vi "Errors Handle Dialoge.vi"(4 ">0, AutoClose":u32, 5 "VI Ref":refnum<vi>, 6 "Cancel Text":string="Cancel", 7 "OK Text":string="OK", 8 "error in (no error)":errorcluster, 9 "DisplayDialog":bool, 10 "Title Text":string, 11 "Message":string="\n\r") -> (0 "error out":errorcluster, 2 "OK?":bool=TRUE)   [LabVIEW 2021]
doc: "Name: 蒋松\nEmail: jiangsong@outlook.com"
uses:
  <userlib>/sushu/Tools/Front Panel State.ctl
panel:
  in  "CloseCounter":string
  in  "Cancel":bool
  in  "OK":bool
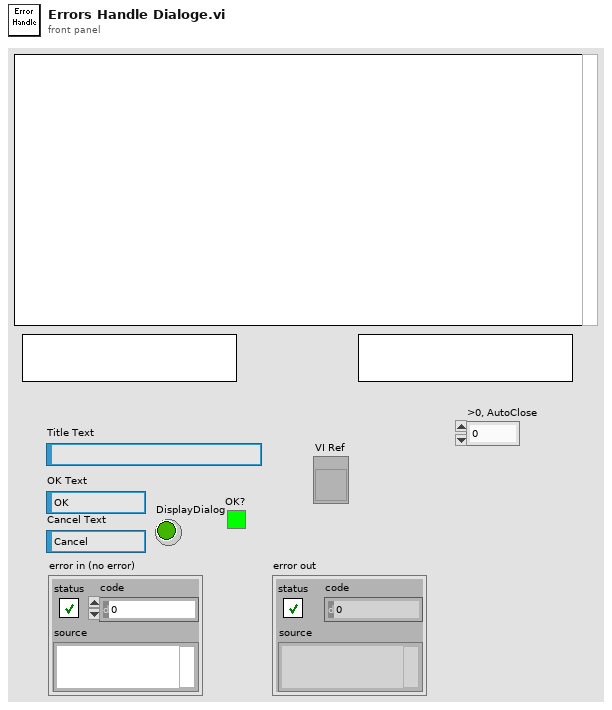
[diagram p1: front panel]
types:
  T1 = typedef "Front Panel State.ctl" = string
  T2 = enum32{"Invalid", "Default", "Floating", "Floating/Auto-Hide", "Modal"}
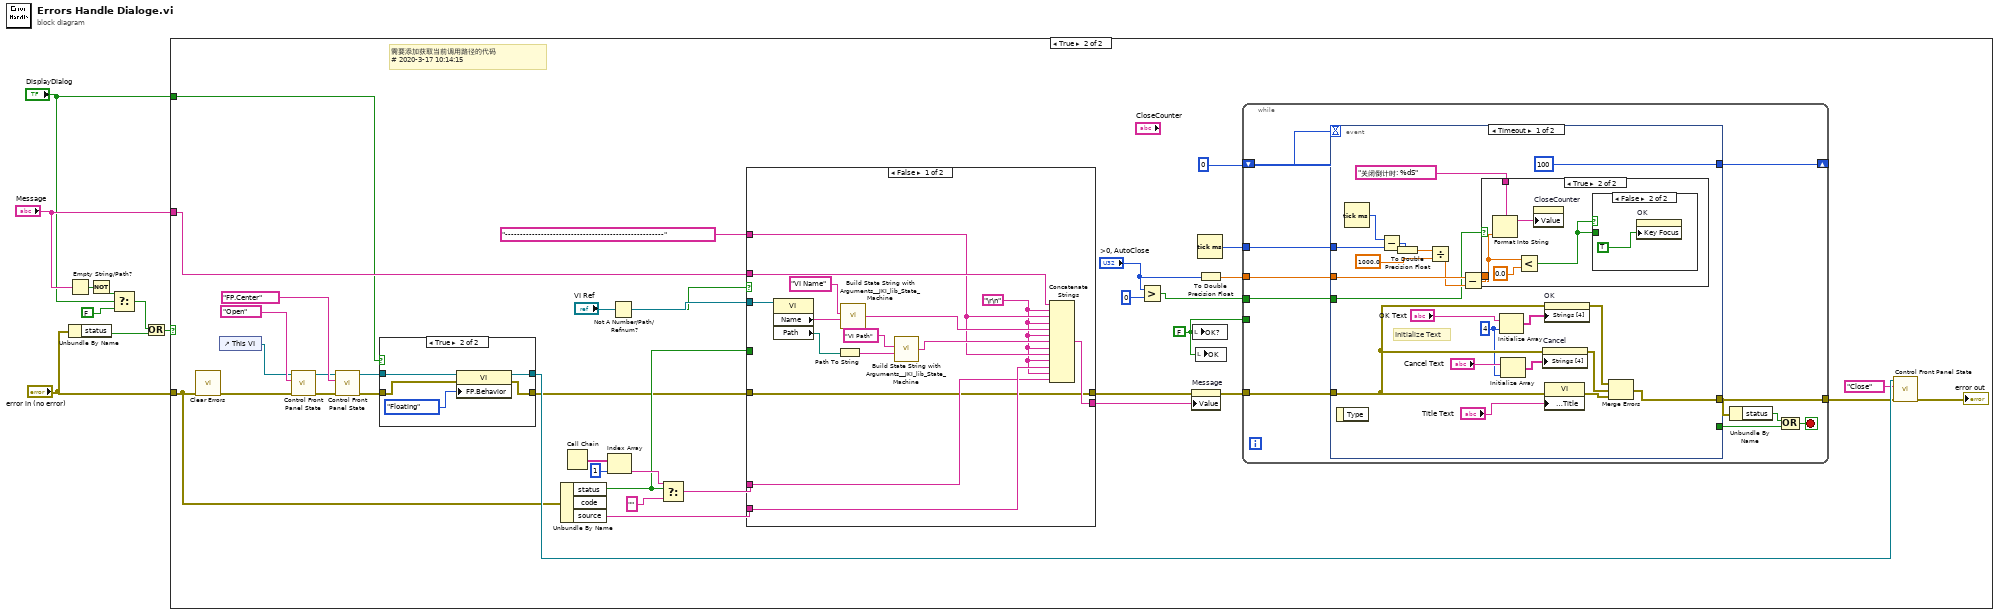
[diagram p0: block diagram]
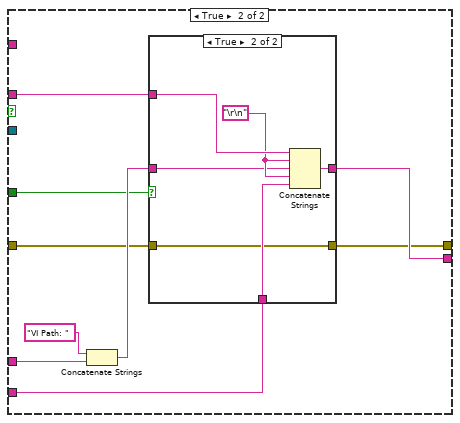
[diagram p4: hidden frame]
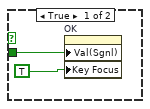
[diagram p7: hidden frame]
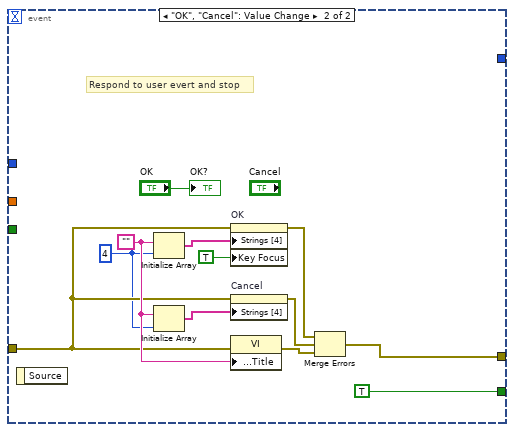
[diagram p8: hidden frame]
diagram:
  n1 = Empty String/Path?(string/path="Message") -> (empty?=w5:bool)
  n2 = Unbundle By Name("error in (no error)") -> ("status"=w9:bool)
  n3 = Not(x=w5) -> (.not. x?=w3:bool)
  n4 = Select(t=w3, s="DisplayDialog", f=FALSE) -> (s? t:f=w4:bool)
  n5 = Or(x=w4, y=w9) -> (x .or. y?=w8:bool)
  n6 = case shown="True" w8 {
    tunnel: "error in (no error)" -> [_ w29]
    tunnel: "Message" -> [_ w34]
    tunnel: "DisplayDialog" -> [_ w30]
    frame False {
    }
    frame True {
      w11 = FALSE ("OK?")
      # "需要添加获取当前调用路径的代码\n# 2020-3-17 10:14:15"
      n7 = call <vilib>:"Clear Errors.vi"("error in (no error)"=w29) -> ("error out"=w28:errorcluster)  [unwired: 5 in, 1 out]
      n8 = control-ref of="This VI"() -> (w26:refnum<vi>)
      n9 = call <userlib>:"Control Front Panel State.vi"("error out"=w28, "Argument"=T1 "Open", "Core.Current VI Reference"=w26) -> ("error out"=w40:errorcluster, "reference out"=w27:refnum<vi>)  [unwired: 7 in]
      n10 = call <userlib>:"Control Front Panel State.vi"("error out"=w40, "Argument"=T1 "FP.Center", "Core.Current VI Reference"=w27) -> ("error out"=w24:errorcluster, "reference out"=w25:refnum<vi>)  [unwired: 7 in]
      n11 = case shown="True" w30 {
        tunnel: w25 -> [w47 w52]
        tunnel: [w47 w50] -> w31
        tunnel: w24 -> [w46 w49]
        tunnel: [w46 w48] -> w23
        frame False {
        }
        frame True {
          n12 = property class="VI"(reference=w52, error in=w49, "FP.Behavior"=T2."Floating" ("Front Panel Window:Behavior")) -> (reference out=w50:refnum<vi>, error out=w48:errorcluster)
        }
      }
      n13 = Unbundle By Name(w29) -> ("status"=w32:bool, "source"=w39:string)  [unwired: 1 out]
      n14 = Call Chain() -> (call chain=w37:string[])
      n15 = Index Array(array=w37, index=1) -> (element=w35:string)
      n16 = Not A Number/Path/Refnum?(number/path/refnum="VI Ref") -> (NaN/Path/Refnum?=w43:bool)
      n17 = Select(t=w35, s=w32, f="") -> (s? t:f=w38:string)
      n18 = case shown="False" w43 {
        tunnel: [w55 w68] -> w22
        tunnel: "VI Ref" -> [w60 _]
        tunnel: w34 -> [w57 w76]
        tunnel: w39 -> [w59 w74]
        tunnel: w38 -> [w58 w75]
        tunnel: w32 -> [_ w71]
        tunnel: w23 -> [w55 w70]
        tunnel: [w56 w69] -> w21
        tunnel: "-----------------------------------------------------" ("string") -> [w54 _]
        frame False {
          w53 = "\r\n"
          n19 = property class="VI"(reference=w60) -> ("Name"=w65:string, "Path"=w67:path)  [unwired: 1 in, 2 out]
          n20 = Path To String(path=w67) -> (string=w62:string)
          n21 = call <vilib>:"Build State String with Arguments__JKI_lib_State_Machine.vi"("Arguments (\"\")"=w65, "State"="VI Name") -> ("State with Arguments"=w64:string)  [unwired: 4 in]
          n22 = call <vilib>:"Build State String with Arguments__JKI_lib_State_Machine.vi"("Arguments (\"\")"=w62, "State"="VI Path") -> ("State with Arguments"=w61:string)  [unwired: 4 in]
          n23 = Concatenate Strings(w57, w53, w54, w53, w64, w53, w61, w53, w54, w53, w59, w53, w58) -> (w56:string)
        }
        frame True {
          n24 = Concatenate Strings("VI Path: " ("string"), w75) -> (w73:string)
          n25 = case shown="True" w71 {
            tunnel: [w78 w84] -> w69
            tunnel: w76 -> [w78 w83]
            tunnel: w74 -> [_ w81]
            tunnel: w73 -> [_ w80]
            tunnel: [w77 w79] -> w68
            tunnel: w70 -> [w77 w79]
            frame False {
            }
            frame True {
              w82 = "\r\n"
              n26 = Concatenate Strings(w83, w82, w80, w82, w81) -> (w84:string)
            }
          }
        }
      }
      n27 = Greater?(x=">0, AutoClose", y=u32 0) -> (0:w12:bool)
      n28 = property on="Message" class="Str"(error in=w22, "Value"=w21) -> (error out=w17:errorcluster)  [unwired: 1 in, 1 out]
      n29 = local write "OK?"(w11) -> ()
      n30 = local write "OK"(w11) -> ()
      n31 = Tick Count (ms)() -> (millisecond timer value=w16:u32)
      n32 = To Double Precision Float(number=">0, AutoClose") -> (double precision float=w13:dbl)
      n33 = while {
        tunnel: w17 -> [w92]
        tunnel: [w91] -> w18
        shift-right: [w93] -> _
        shift-left: 0 -> [w94]
        tunnel: w16 -> [w87]
        tunnel: w13 -> [w86]
        tunnel: w12 -> [w85]
        tunnel: w11 -> [_]
        stop <- w88 stop-if-true
        n34 = event shown="[0] Timeout" {
          selector: _ -> [_ _]
          dyn-events: _ -> [_ _]
          timeout: w94 -> [_ _]
          tunnel: [100 _] -> w93
          tunnel: w92 -> [w111 w128]
          tunnel: [w114 w134] -> w91
          tunnel: [_ TRUE] -> w89
          tunnel: w87 -> [w103 _]
          tunnel: w86 -> [w102 _]
          tunnel: w85 -> [w95 _]
          event Timeout {
            w107 = 4 ("dimension size")
            # "Initialize Text"
            n35 = event-data() -> ()  [unwired: 1 in, 1 out]
            n36 = Tick Count (ms)() -> (millisecond timer value=w104:u32)
            n37 = Subtract(x=w104, y=w103) -> (x-y=w101:u32)
            n38 = To Double Precision Float(number=w101) -> (double precision float=w97:dbl)
            n39 = Divide(x=w97, y=1000.0) -> (x/y=w99:dbl)
            n40 = Subtract(x=w102, y=w99) -> (x-y=w96:dbl)
            n41 = case shown="True" w95 {
              tunnel: "关闭倒计时: %dS" ("CloseCounter") -> [_ w121]
              tunnel: w96 -> [_ w119]
              frame False {
              }
              frame True {
                n42 = Format Into String(format string=w121, w119) -> (resulting string=w120:string)  [unwired: 2 in, 1 out]
                n43 = Less?(x=w119, y=0.0) -> (x < y?=w117:bool)
                n44 = property on="CloseCounter" class="Str"("Value"=w120) -> ()  [unwired: 2 in, 2 out]
                n45 = case shown="False" w117 {
                  tunnel: w117 -> [w123 _]
                  frame True {
                    n46 = property on="OK" class="Bool (strict)"("Val(Sgnl)"=w123, "Key Focus"=TRUE) -> ()  [unwired: 2 in, 2 out]
                  }
                  frame False {
                    n47 = property on="OK" class="Bool (strict)"("Key Focus"=TRUE) -> ()  [unwired: 2 in, 2 out]
                  }
                }
              }
            }
            n48 = Initialize Array("OK Text", w107) -> (w108:string[])
            n49 = Initialize Array("Cancel Text", w107) -> (w106:string[])
            n50 = property on="Cancel" class="Bool"(error in=w111, "Strings [4]"=w106) -> (error out=w113:errorcluster)  [unwired: 1 in, 1 out]
            n51 = property on="OK" class="Bool (strict)"(error in=w111, "Strings [4]"=w108) -> (error out=w112:errorcluster)  [unwired: 1 in, 1 out]
            n52 = property class="VI"(error in=w111, "Front Panel.Title"="Title Text") -> (error out=w115:errorcluster)  [unwired: 1 in, 1 out]
            n53 = Merge Errors(w112, w113, w115) -> (w114:errorcluster)
          }
          event "OK", "Cancel": Value Change {
            w125 = 4 ("dimension size")
            w129 = ""
            # "Respond to user evert and stop"
            n54 = event-data() -> ()  [unwired: 1 in, 1 out]
            n55 = Initialize Array(w129, w125) -> (w130:string[])
            n56 = Initialize Array(w129, w125) -> (w131:string[])
            n57 = property on="OK" class="Bool (strict)"(error in=w128, "Strings [4]"=w130, "Key Focus"=TRUE) -> (error out=w132:errorcluster)  [unwired: 1 in, 1 out]
            n58 = property on="Cancel" class="Bool"(error in=w128, "Strings [4]"=w131) -> (error out=w133:errorcluster)  [unwired: 1 in, 1 out]
            n59 = property class="VI"(error in=w128, "Front Panel.Title"=w129) -> (error out=w135:errorcluster)  [unwired: 1 in, 1 out]
            n60 = Merge Errors(w132, w133, w135) -> (w134:errorcluster)
            "OK?" <- "OK"
          }
        }
        n61 = Unbundle By Name(w91) -> ("status"=w90:bool)
        n62 = Compound Arithmetic op=OR(w90, w89) -> (w88:bool)
      }
      n63 = call <userlib>:"Control Front Panel State.vi"("error out"=w18, "Argument"=T1 "Close", "Core.Current VI Reference"=w31) -> ("error out"=→"error out":errorcluster)  [unwired: 7 in, 1 out]
    }
  }
